vi "Logging Stopped.vi"(8 "error in (no error)":errorcluster) -> (0 "error out":errorcluster)   [LabVIEW 2014, in "Logger.lvlib"]
uses:
  Logger.lvlib
  Stop Logging Argument--cluster.ctl
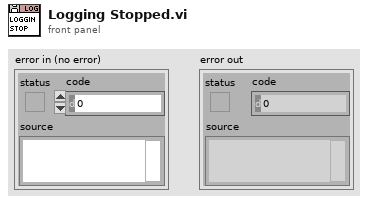
[diagram p1: front panel]
types:
  T1 = typedef "Logger.lvlib/Stop Logging Argument--cluster.ctl" = cluster{"Boolean":bool}
  T2 = typedef "Logger.lvlib/Broadcast Events--cluster.ctl" = cluster{"Module Did Init":refnum<user-event>, "Status Updated":refnum<user-event>, "Error Reported":refnum<user-event>, "Module Did Stop":refnum<user-event>, "Update Module Execution Status":refnum<user-event>, "Logging Stopped":refnum<user-event>, "File Initialized":refnum<user-event>}
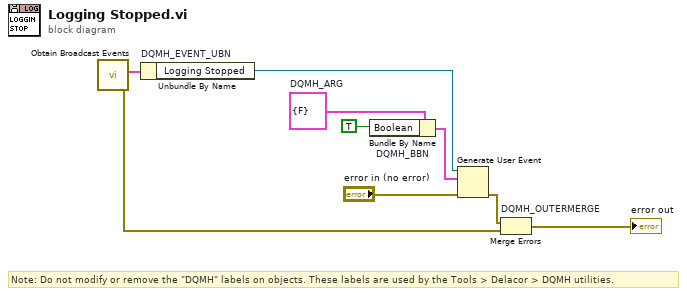
[diagram p0: block diagram]
diagram:
  w4 = T1 {"Boolean"=FALSE}  # DQMH_ARG
  # "Note: Do not modify or remove the \"DQMH\" labels on objects. These labels are used by the Tools > Delacor > DQMH utilities."
  n1 = call "Obtain Broadcast Events.vi"() -> ("error out"=w2:errorcluster, "Logger Broadcast Events"=w1:T2)  [unwired: 10 in]
  n2 = Unbundle By Name "DQMH_EVENT_UBN"(w1) -> ("Logging Stopped"=w6:refnum<user-event>)
  n3 = Bundle By Name "DQMH_BBN"(cluster=w4, "Boolean"=TRUE) -> (w7:T1)
  n4 = Generate User Event(user event=w6, event data cluster=w7, error in="error in (no error)") -> (error out=w5:errorcluster)  [unwired: 1 in, 1 out]
  n5 = Merge Errors "DQMH_OUTERMERGE"(w5, w2) -> (→"error out":errorcluster)
